vi "Set Fit Plot Properties.vi"(6 "Fit array start":i32=2, 8 "error in (no error)":errorcluster, 9 "Good fit?":dbl[](array[numeric])=[1.0] format="%#_4p", 10 "Fit array size":i32, 11 "Resonance Detector in":refnum<class "Resonance Detector.lvclass">) -> (0 "error out":errorcluster, 3 "Resonance Detector out":refnum<class "Resonance Detector.lvclass">)   [LabVIEW 2020, in "Resonance Detector.lvclass"]
uses:
  Resonance Detector.lvclass
  Resonance Detector.lvclass/Resonance Detector.ctl
  d9744acf-01e8-4c96-a561-db65a0164af1.vi
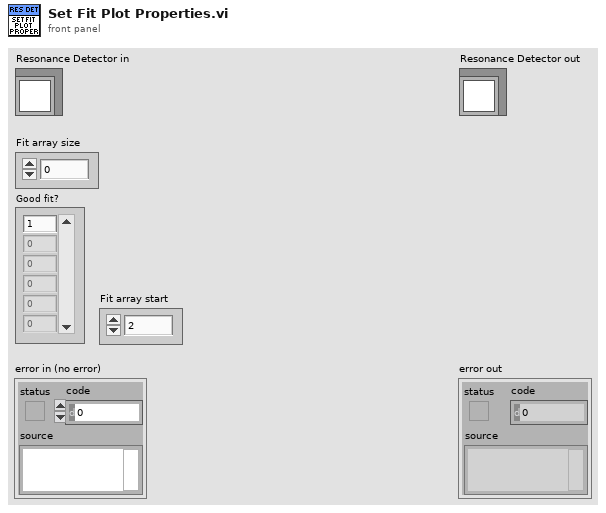
[diagram p1: front panel]
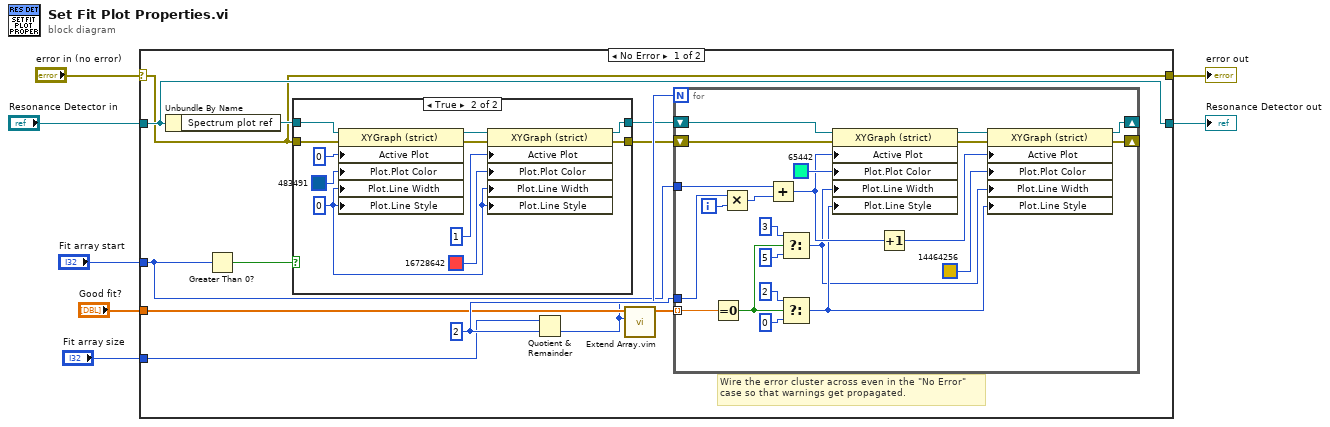
[diagram p0: block diagram]
diagram:
  n1 = case shown="No Error" "error in (no error)" {
    selector: "error in (no error)" -> [w10 w56]
    tunnel: [w10 w56] -> w6
    tunnel: [w19 w55] -> w4
    tunnel: "Resonance Detector in" -> [w19 w55]
    tunnel: "Fit array size" -> [w17 _]
    tunnel: "Good fit?" -> [w16 _]
    tunnel: "Fit array start" -> [w13 _]
    frame No Error {
      w18 = 2 ("y")
      # "Wire the error cluster across even in the \"No Error\"\ncase so that warnings get propagated."
      n2 = Unbundle By Name(w19) -> ("Spectrum plot ref"=w11:refnum<vi>)
      n3 = Greater Than 0?(x=w13) -> (x > 0?=w12:bool)
      n4 = case shown="True" w12 {
        tunnel: w11 -> [w20 w26]
        tunnel: w10 -> [w21 w25]
        tunnel: [w21 w24] -> w9
        tunnel: [w20 w23] -> w8
        frame False {
        }
        frame True {
          w27 = u8 0 ("Plot.Line Width")
          n5 = property class="XYGraph (strict)"(reference=w26, error in=w25, "Active Plot"=u32 0, "Plot.Plot Color"=u32 483491, "Plot.Line Width"=w27, "Plot.Line Style"=w27) -> (reference out=w31:refnum<vi>, error out=w32:errorcluster)
          n6 = property class="XYGraph (strict)"(reference=w31, error in=w32, "Active Plot"=u32 1, "Plot.Plot Color"=u32 16728642, "Plot.Line Width"=w27, "Plot.Line Style"=w27) -> (reference out=w23:refnum<vi>, error out=w24:errorcluster)
        }
      }
      n7 = Quotient & Remainder(x=w17, y=w18) -> (floor(x/y)=w15:i32)  [unwired: 1 out]
      n8 = call "Extend Array.vim"("Extend to size"=w15, "Array in"=w16) -> ("Array out"=w14:dbl[])  [unwired: 8 in, 1 out]
      n9 = for {
        N: w15 -> [_]
        shift-right: [w45] -> _
        shift-left: w9 -> [w53]
        shift-right: [w44] -> _
        shift-left: w8 -> [w54]
        tunnel: w18 -> [w42]
        tunnel: w14 -> [w41] mode=indexing
        tunnel: w13 -> [w33]
        i -> [w52]
        n10 = Equal To 0?(x=w41) -> (x = 0?=w35:bool)
        n11 = Multiply(x=w42, y=w52) -> (x*y=w43:i32)
        n12 = Add(x=w33, y=w43) -> (x+y=w48:i32)
        n13 = Select(t=u8 3 ("Plot.Line Width"), s=w35, f=u8 5 ("Plot.Line Width")) -> (s? t:f=w34:u8)
        n14 = Select(t=u8 2, s=w35, f=u8 0 ("Plot.Line Style")) -> (s? t:f=w39:u8)
        n15 = property class="XYGraph (strict)"(reference=w54, error in=w53, "Active Plot"=w48, "Plot.Plot Color"=u32 65442 ("Color Box"), "Plot.Line Width"=w34, "Plot.Line Style"=w39) -> (reference out=w50:refnum<vi>, error out=w49:errorcluster)
        n16 = Increment(x=w48) -> (x+1=w47:i32)
        n17 = property class="XYGraph (strict)"(reference=w50, error in=w49, "Active Plot"=w47, "Plot.Plot Color"=u32 14464256 ("Color Box"), "Plot.Line Width"=w34, "Plot.Line Style"=w39) -> (reference out=w44:refnum<vi>, error out=w45:errorcluster)
      }
    }
    frame Error {
    }
  }
  "error out" <- w6
  "Resonance Detector out" <- w4
